vi "属性节点（Labview真好用！）.vi"() -> ()   [LabVIEW 2017]
panel:
  out "字符串":string
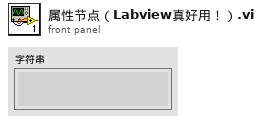
[diagram p1: front panel]
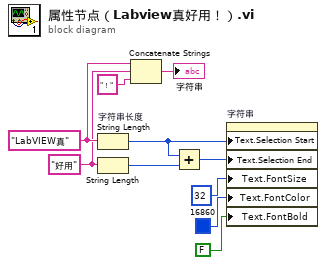
[diagram p0: block diagram]
diagram:
  w7 = "好用"
  w8 = "LabVIEW真"
  n1 = String Length "字符串长度"(string=w8) -> (length=w5:i32)
  n2 = String Length(string=w7) -> (length=w6:i32)
  n3 = Concatenate Strings(w8, w7, "！") -> (→"字符串":string)
  n4 = Add(x=w5, y=w6) -> (x+y=w4:i32)
  n5 = property on="字符串" class="Str"("Text.Selection Start"=w5, "Text.Selection End"=w4, "Text.FontSize"=u32 32 ("文本.字体:字号"), "Text.FontColor"=u32 16860, "Text.FontBold"=FALSE ("文本.字体:粗体")) -> ()  [unwired: 2 in, 2 out]
